vi "_Raise Script Dialog Opening.vi"(4 "WebView2.lvlib:WebView2 Control.lvclass":refnum<class "WebView2 Control.lvclass">, 5 "Event Data":cluster{"sender":refnum<k24>, "e":refnum<k24>}, 6 "Control Ref":refnum<k24>, 7 "Event Common Data":T1) -> ()   [LabVIEW 2025, in "WebView2.lvlib" / "WebView2 Control.lvclass"]
uses:
  WebView2 Control.lvclass
  WebView2 Control.lvclass/WebView2 Control.ctl
  E:/Labview/LV 2023/PPL/PPL Builder/Libs/LV-WebView2/Source/Libs/Microsoft.Web.WebView2.Core.dll
  Libs/Microsoft.Web.WebView2.Core.dll
  Script Dialog Opening Event Data.ctl
  WebView2 Event Filter Interface/WebView2 Event Filter Interface.lvclass
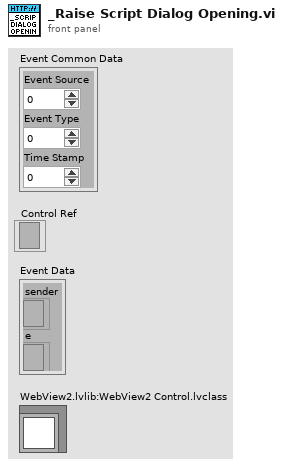
[diagram p1: front panel]
types:
  T1 = cluster{"Event Source":i32, "Event Type":u32, "Time Stamp":u32}
  T2 = typedef "WebView2.lvlib/WebView2 Control.lvclass/Script Dialog Opening Event Data.ctl" = cluster{"DefaultText":string, "Kind":i32, "Message":string, "Uri":string}
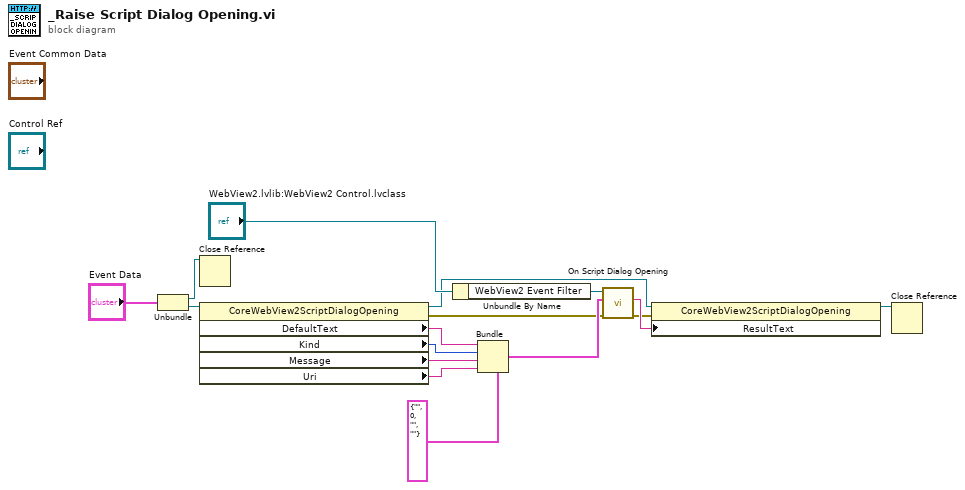
[diagram p0: block diagram]
diagram:
  n1 = Unbundle("Event Data") -> ("sender"=w15:refnum<k24>, "e"=w14:refnum<k24>)
  n2 = Close Reference(reference=w15) -> ()  [unwired: 1 in, 1 out]
  n3 = property class="CoreWebView2ScriptDialogOpening"(reference=w14) -> (reference out=w4:refnum<k24>, error out=w5:errorcluster, "DefaultText"=w13:string, "Kind"=w12:i32, "Message"=w11:string, "Uri"=w10:string)  [unwired: 1 in]
  n4 = Unbundle By Name("WebView2.lvlib:WebView2 Control.lvclass") -> ("WebView2 Event Filter"=w6:refnum<class "WebView2 Event Filter Interface.lvclass">)
  n5 = Bundle(cluster=T2 {"DefaultText"="", "Kind"=0, "Message"="", "Uri"=""}, "DefaultText"=w13, "Kind"=w12, "Message"=w11, "Uri"=w10) -> (w8:T2)
  n6 = call-dynamic "On Script Dialog Opening.vi"("error in (no error)"=w5, "Data"=w8, "WebView2 Event Filter Interface in"=w6) -> ("error out"=w2:errorcluster, "ResultText"=w3:string)  [unwired: 7 in]
  n7 = property class="CoreWebView2ScriptDialogOpening"(reference=w4, error in=w2, "ResultText"=w3) -> (reference out=w1:refnum<k24>)  [unwired: 1 out]
  n8 = Close Reference(reference=w1) -> ()  [unwired: 1 in, 1 out]
